vi "Buy Action.vi"(8 "error in (no error)":errorcluster, 11 "Stock Trader In":refnum<class "Stock Trader.lvclass">) -> (0 "error out":errorcluster, 3 "Stock Trader Out":refnum<class "Stock Trader.lvclass">)   [LabVIEW 2019, in "Stock Trader.lvclass"]
doc: "Executes a Buy Action. This is where Stock Trader, the receiver, processes the Buy Stock Order concrete command. Called from the Buy Stock Order Execute override."
uses:
  Stock Trader.lvclass
  Stock Trader.lvclass/Stock Trader.ctl
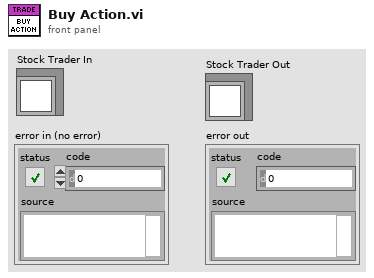
[diagram p1: front panel]
types:
  T1 = typedef "Display Event.ctl" = refnum<user-event>
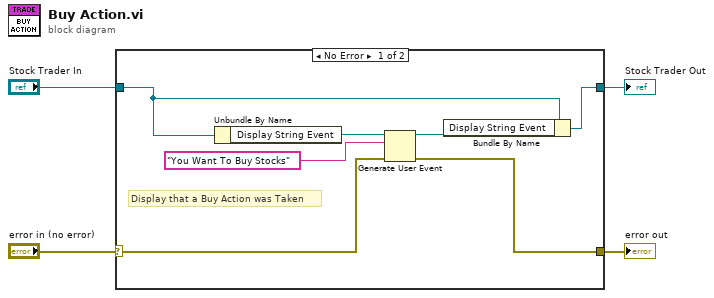
[diagram p0: block diagram]
diagram:
  n1 = case shown="No Error" "error in (no error)" {
    selector: "error in (no error)" -> [w9 w13]
    tunnel: [w8 w13] -> w3
    tunnel: "Stock Trader In" -> [w6 w12]
    tunnel: [w5 w12] -> w1
    frame No Error {
      # "Display that a Buy Action was Taken"
      n2 = Unbundle By Name(w6) -> ("Display String Event"=w11:T1)
      n3 = Generate User Event(user event=w11, event data cluster="You Want To Buy Stocks" ("event data"), error in=w9) -> (user event out=w7:T1, error out=w8:errorcluster)  [unwired: 1 in]
      n4 = Bundle By Name(cluster=w6, "Display String Event"=w7) -> (w5:refnum<class "Stock Trader.lvclass">)
    }
    frame Error {
    }
  }
  "error out" <- w3
  "Stock Trader Out" <- w1
